vi "Unscramble All Global Fit Plots.vi"(6 "Residual Type":T1, 7 "# Points in Plots":i32[](array[numeric]), 8 "Error In":errorcluster, 9 "Best Nonlinear Fit Array":dbl[](array[numeric]), 10 "Y array":dbl[](array[numeric]), 11 "t Array":dbl[](array[numeric])) -> (0 "Error Out":errorcluster, 1 "Decay Residuals":cluster{"Array":dbl[], "Array":dbl[]}[](array[cluster]), 3 "Fitted Decays":cluster{"Array":dbl[], "Array":dbl[]}[](array[cluster]))   [LabVIEW 2021, in "AlliGator Global Decay Fit.lvlib"]
uses:
  Residual Type.ctl
  AlliGator/AlliGator Global Decay Fit.lvlib
  Fits.lvlib
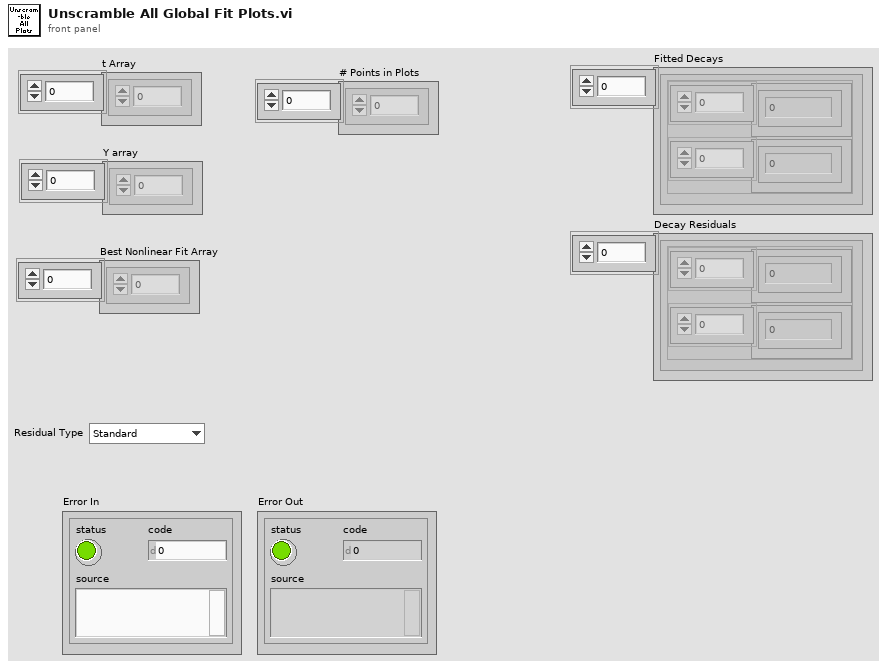
[diagram p1: front panel]
types:
  T1 = typedef "Fits.lvlib/Residual Type.ctl" = enum16{"Standard", "Normalized", "Reduced"}
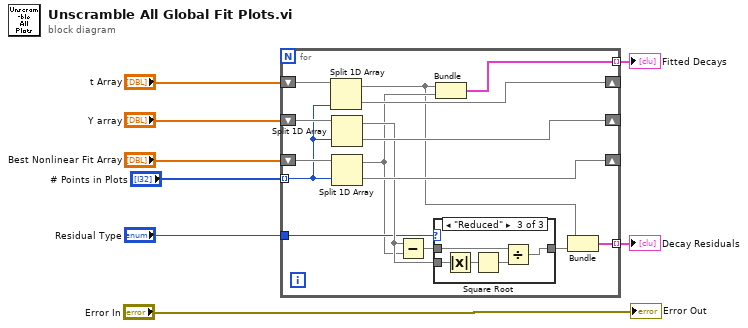
[diagram p0: block diagram]
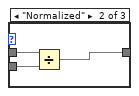
[diagram p3: hidden frame]
diagram:
  n1 = for {
    tunnel: "# Points in Plots" -> [w20] mode=indexing
    shift-right: [w19] -> _
    shift-left: "t Array" -> [w23]
    shift-right: [w18] -> _
    shift-left: "Y array" -> [w22]
    shift-right: [w17] -> _
    shift-left: "Best Nonlinear Fit Array" -> [w21]
    tunnel: "Residual Type" -> [w14]
    tunnel: [w12] -> w4 mode=indexing
    tunnel: [w9] -> w3 mode=indexing
    n2 = Split 1D Array(array=w23, index=w20) -> (first subarray=w10:dbl[], second subarray=w19:dbl[])
    n3 = Split 1D Array(array=w22, index=w20) -> (first subarray=w15:dbl[], second subarray=w18:dbl[])
    n4 = Split 1D Array(array=w21, index=w20) -> (first subarray=w13:dbl[], second subarray=w17:dbl[])
    n5 = Subtract(x=w15, y=w13) -> (x-y=w16:dbl[])
    n6 = case shown="\"Reduced\"" w14 {
      tunnel: w16 -> [w24 w27 w32]
      tunnel: [w24 w25 w30] -> w11
      tunnel: w15 -> [_ w26 w31]
      frame "Standard", Default {
      }
      frame "Normalized" {
        n7 = Divide(x=w27, y=w26) -> (x/y=w25:dbl[])
      }
      frame "Reduced" {
        n8 = Absolute Value(x=w31) -> (abs(x)=w29:dbl[])
        n9 = Square Root(x=w29) -> (sqrt(x)=w28:dbl[])
        n10 = Divide(x=w32, y=w28) -> (x/y=w30:dbl[])
      }
    }
    n11 = Bundle(w10, w13) -> (w12:cluster{dbl[], dbl[]})  [unwired: 1 in]
    n12 = Bundle(w10, w11) -> (w9:cluster{dbl[], dbl[]})  [unwired: 1 in]
  }
  "Fitted Decays" <- w4
  "Decay Residuals" <- w3
  "Error Out" <- "Error In"
